vi "QCP_Get.vi"   [LabVIEW 2016]
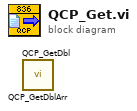
[diagram p0: block diagram]
diagram:
  n1 = call <userlib>:"QCP_GetDblArr.vi"() -> ()  [unwired: 9 in, 3 out]
  n2 = call <userlib>:"QCP_GetDbl.vi"() -> ()  [unwired: 9 in, 3 out]
